vi "16bit Image Normalization.vi"(8 "Transpose":bool=TRUE, 10 "Imput image bits":u8=16, 11 "Input image":i16[][](graph)) -> (0 "min":i16, 1 "mean":i16, 2 "max":i16, 3 "Normalized image":u8[][](graph), 5 "Direct scaled image":u8[][](graph))   [LabVIEW 2018]
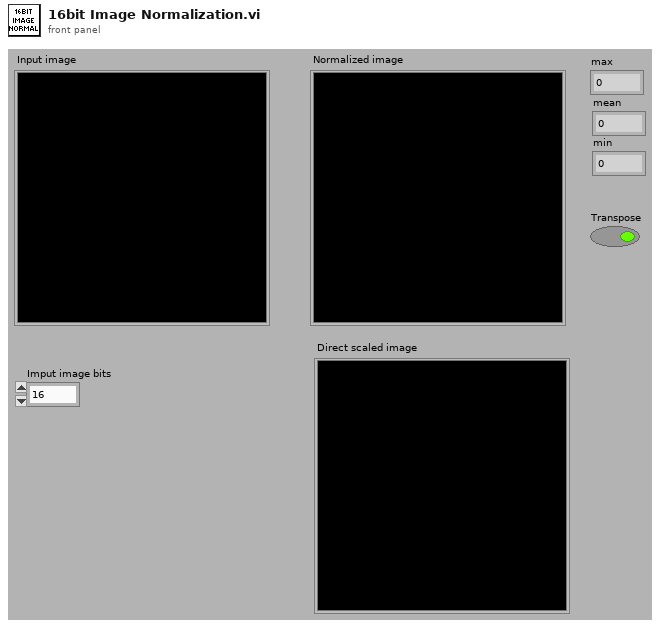
[diagram p1: front panel]
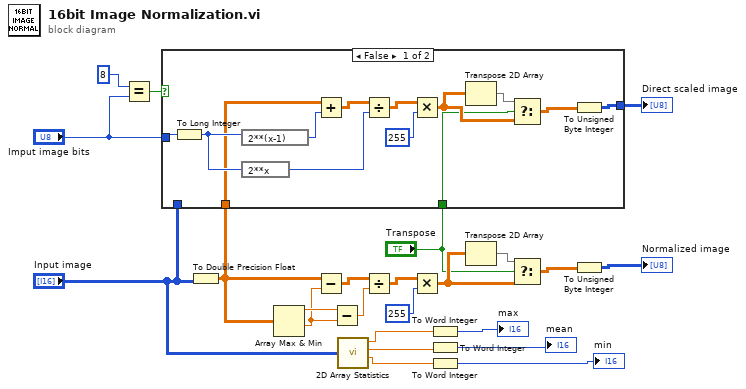
[diagram p0: block diagram]
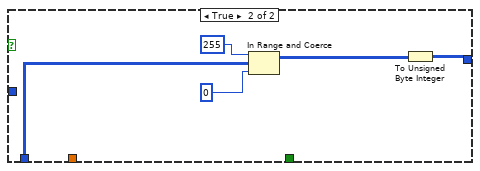
[diagram p2: hidden frame]
diagram:
  n1 = Equal?(x=u8 8, y="Imput image bits") -> (x = y?=w4:bool)
  n2 = To Double Precision Float(number="Input image") -> (double precision float=w5:dbl[][])
  n3 = case shown="False" w4 {
    tunnel: [w31 w41] -> w7
    tunnel: "Transpose" -> [w29 _]
    tunnel: "Imput image bits" -> [w28 _]
    tunnel: w5 -> [w24 _]
    tunnel: "Input image" -> [_ w40]
    frame False {
      n4 = To Long Integer(number=w28) -> (32bit integer=w25:i32)
      n5 = expression code="2**(x-1)"(w25) -> (w26:i32)
      n6 = expression code="2**x"(w25) -> (w27:i32)
      n7 = Add(x=w24, y=w26) -> (x+y=w34:dbl[][])
      n8 = Divide(x=w34, y=w27) -> (x/y=w35:dbl[][])
      n9 = Multiply(x=w35, y=255) -> (x*y=w30:dbl[][])
      n10 = Transpose 2D Array(2D array=w30) -> (transposed array=w33:dbl[][])
      n11 = Select(t=w33, s=w29, f=w30) -> (s? t:f=w32:dbl[][])
      n12 = To Unsigned Byte Integer(number=w32) -> (unsigned 8bit integer=w31:u8[][])
    }
    frame True {
      n13 = In Range and Coerce(upper limit=u8 255 ("x"), x=w40, lower limit=u8 0 ("x")) -> (coerced(x)=w38:i16[][])  [unwired: 1 out]
      n14 = To Unsigned Byte Integer(number=w38) -> (unsigned 8bit integer=w41:u8[][])
    }
  }
  "Direct scaled image" <- w7
  n15 = Array Max & Min(array=w5) -> (max value=w19:dbl, min value=w18:dbl)  [unwired: 2 out]
  n16 = Subtract(x=w5, y=w18) -> (x-y=w20:dbl[][])
  n17 = Subtract(x=w19, y=w18) -> (x-y=w17:dbl)
  n18 = call "2D Array Statistics.vi"("array"="Input image") -> ("max"=w21:dbl, "mean"=w22:dbl, "min"=w23:dbl)  [unwired: 5 out]
  n19 = Divide(x=w20, y=w17) -> (x/y=w16:dbl[][])
  n20 = Multiply(x=w16, y=255) -> (x*y=w8:dbl[][])
  n21 = To Word Integer(number=w21) -> (16bit integer=→"max":i16)
  n22 = To Word Integer(number=w22) -> (16bit integer=→"mean":i16)
  n23 = To Word Integer(number=w23) -> (16bit integer=→"min":i16)
  n24 = Transpose 2D Array(2D array=w8) -> (transposed array=w9:dbl[][])
  n25 = Select(t=w9, s="Transpose", f=w8) -> (s? t:f=w10:dbl[][])
  n26 = To Unsigned Byte Integer(number=w10) -> (unsigned 8bit integer=→"Normalized image":u8[][])
